vi "SERIAL_VerifyChecksum.vi"(1 "Content":string) -> (0 "Valid Checksum":bool)   [LabVIEW 2018, in "navX-MXP IMU.lvlib"]
uses:
  navX-MXP IMU.lvlib
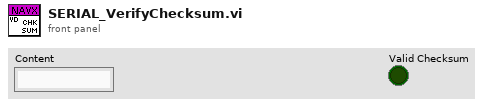
[diagram p1: front panel]
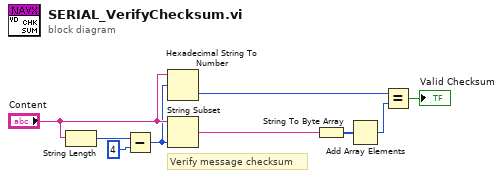
[diagram p0: block diagram]
diagram:
  # "Verify message checksum"
  n1 = String Length(string="Content") -> (length=w9:i32)
  n2 = Subtract(x=w9, y=4) -> (x-y=w4:i32)
  n3 = Hexadecimal String To Number(string="Content", offset=w4) -> (number=w2:u32)  [unwired: 1 in, 1 out]
  n4 = String Subset(string="Content", length (rest)=w4) -> (substring=w6:string)  [unwired: 1 in]
  n5 = String To Byte Array(string=w6) -> (unsigned byte array=w7:u8[])
  n6 = Add Array Elements(numeric array=w7) -> (sum=w3:u8)
  n7 = Equal?(x=w2, y=w3) -> (x = y?=→"Valid Checksum":bool)
